vi "Thermochiller_NEWEST.vi"() -> ()   [LabVIEW 2016]
uses:
  <vilib>/Instr/_visa.llb/VISA Configure Serial Port (Instr).vi
panel:
  in  "flow control (0:none)":u16(ring) items=["None", "XON/XOFF", "RTS/CTS", "XON/XOFF & RTS/CTS", "DTR/DSR", "XON/XOFF & DTR/DSR"]
  in  "stop bits (10: 1 bit)":u16(ring)=10 items=["1.0"=10, "1.5"=15, "2.0"=20]
  in  "parity (0:none)":enum16{"None", "Odd", "Even", "Mark", "Space"}(ring)
  in  "data bits (8)":u16=8
  in  "VISA resource name":refnum<visa-resource-name>
  out "Temperature 3":cluster{"Y":dbl[], "Y":dbl[]}[](graph)
  in  "Exit":bool
  in  "Graph":bool
  out "Read Current T":string
  out "Temperature 2":dbl(knob) scale=0.0..50.0
  out "T, C":dbl
  in  "Set T Button":bool
  in  "Set T":dbl
  # "SMC THERMOCHILLER HRS -"
  # "Конфигурация оборудования"
  # "Установка температуры"
  # "Текущая температура"
  # "(c) 2021 Vladimir Z Inc.  ALL RIGHTS RESERVED."
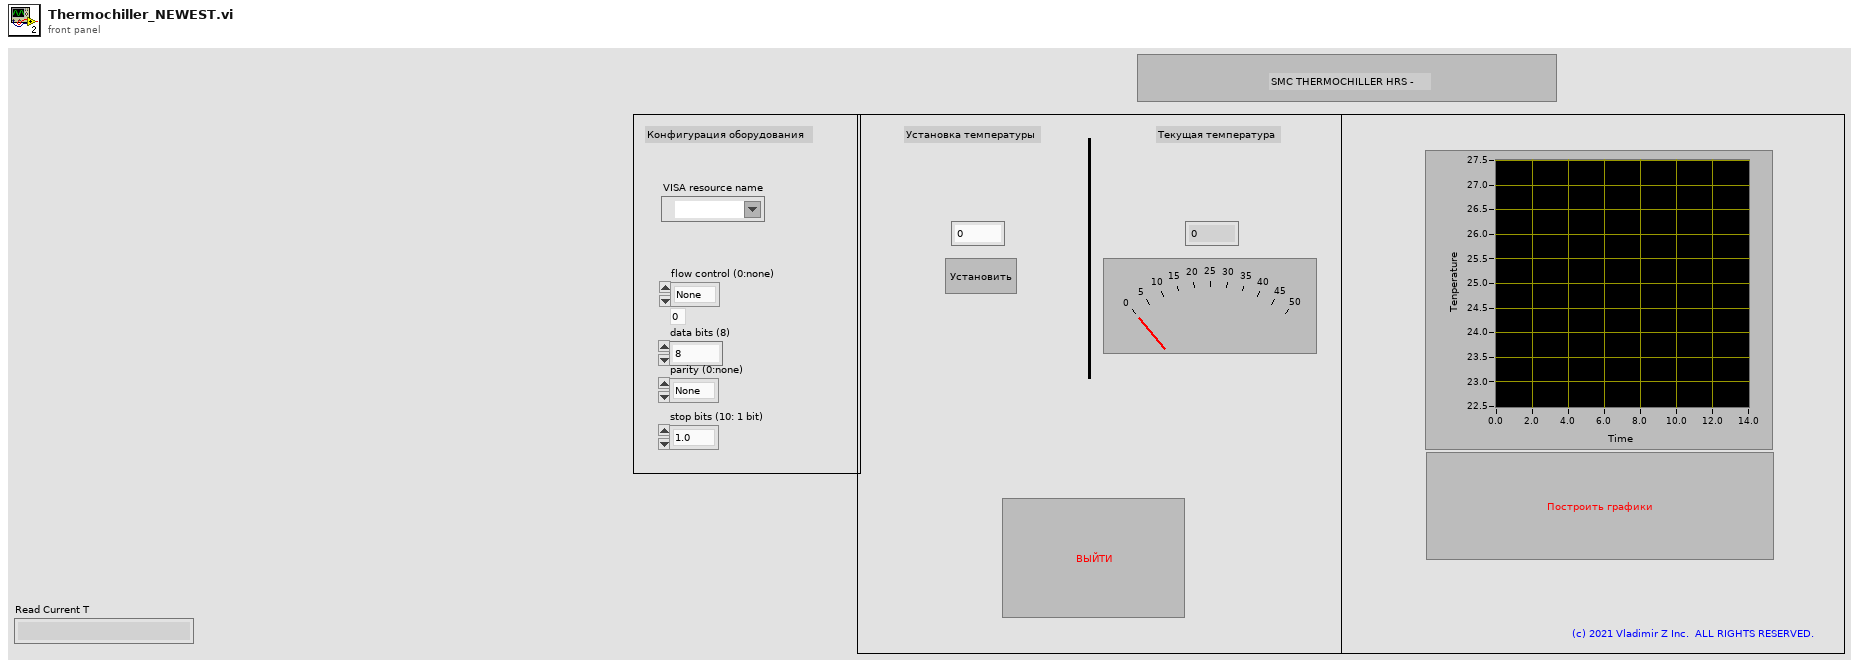
[diagram p1: front panel]
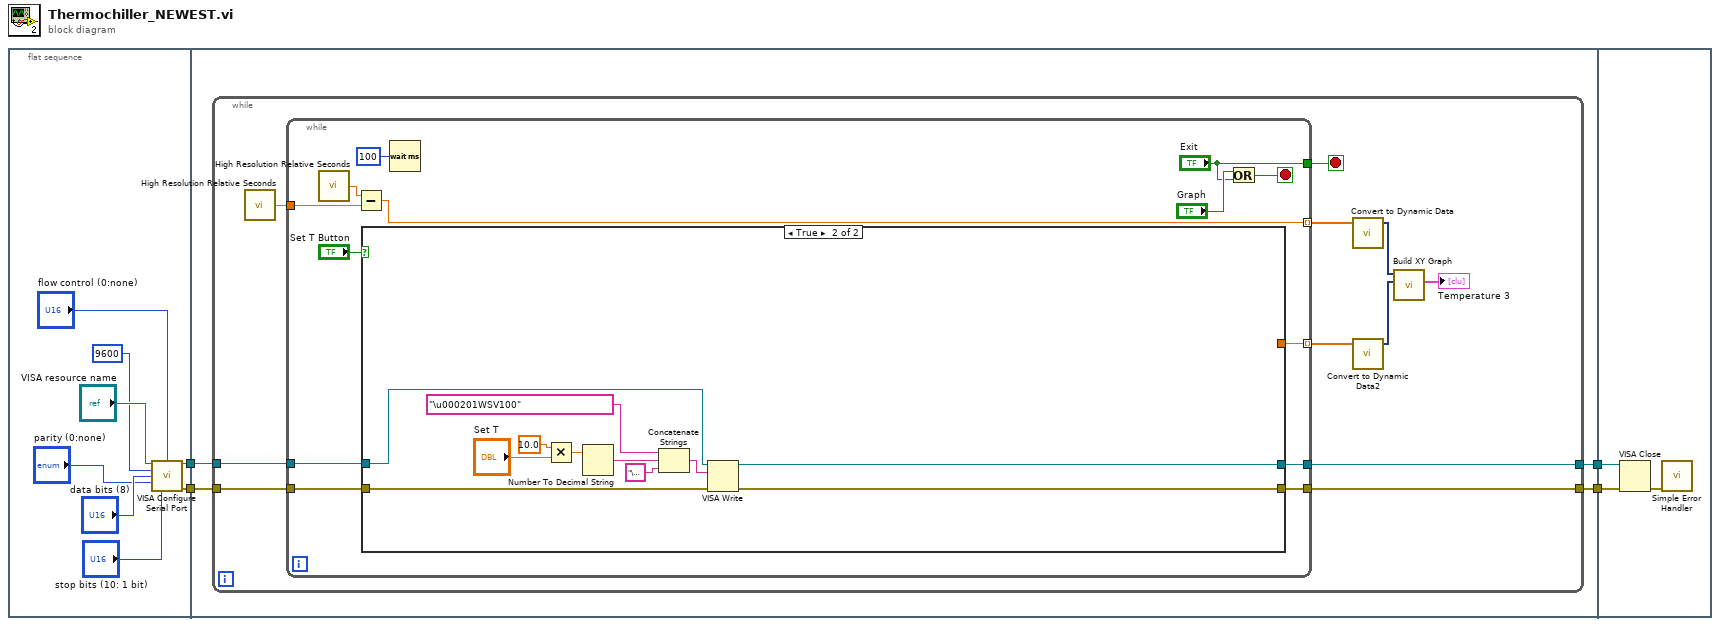
[diagram p0: block diagram]
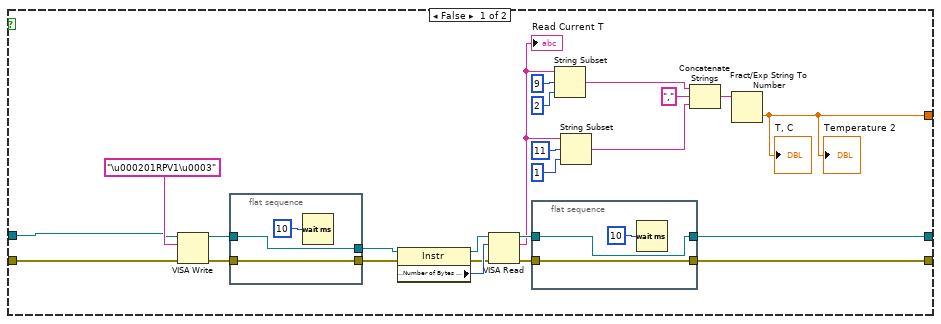
[diagram p2: hidden frame]
diagram:
  n1 = flat-sequence {
    tunnel: [w8] -> w4
    tunnel: [w7] -> w3
    tunnel: w4 -> [w16]
    tunnel: w3 -> [w15]
    tunnel: [w14] -> w2
    tunnel: [w13] -> w1
    tunnel: w2 -> [w84]
    tunnel: w1 -> [w83]
    frame #0 {
      n2 = call-poly "VISA Configure Serial Port"("VISA resource name"="VISA resource name", "baud rate (9600)"=u32 9600, "data bits (8)"="data bits (8)", "parity (0:none)"="parity (0:none)", "stop bits (10: 1 bit)"="stop bits (10: 1 bit)", "flow control (0:none)"="flow control (0:none)") -> ("VISA resource name out"=w8:refnum<visa-resource-name>, "error out"=w7:errorcluster)  [unwired: 8 in]
    }
    frame #1 {
      n3 = while {
        tunnel: w16 -> [w20]
        tunnel: w15 -> [w19]
        tunnel: [w18] -> w14
        tunnel: [w17] -> w13
        stop <- w21 stop-if-true
        n4 = call <vilib>:"High Resolution Relative Seconds.vi"() -> ("relative seconds"=w27:dbl)
        n5 = while {
          tunnel: w27 -> [w38]
          tunnel: [w36] -> w25 mode=indexing
          tunnel: [w35] -> w23 mode=indexing
          tunnel: ["Exit"] -> w21
          tunnel: w20 -> [w32]
          tunnel: w19 -> [w31]
          tunnel: [w30] -> w18
          tunnel: [w29] -> w17
          stop <- w34 stop-if-true
          n6 = call <vilib>:"High Resolution Relative Seconds.vi"() -> ("relative seconds"=w37:dbl)
          n7 = Subtract(x=w37, y=w38) -> (x-y=w36:dbl)
          n8 = case shown="True" "Set T Button" {
            tunnel: [w45 _] -> w35
            tunnel: w32 -> [w44 w74]
            tunnel: w31 -> [w43 w73]
            tunnel: [w42 w72] -> w30
            tunnel: [w41 w71] -> w29
            frame False {
              n9 = VISA Write(VISA resource name=w44, write buffer="\u000201RPV1\u0003", error in (no error)=w43) -> (VISA resource name out=w48:refnum<visa-resource-name>, error out=w49:errorcluster)  [unwired: 1 out]
              n10 = flat-sequence {
                tunnel: [w68] -> w64
                tunnel: [w69] -> w63
                tunnel: w49 -> [w69]
                tunnel: w48 -> [w68]
                frame #0 {
                  n11 = Wait (ms)(milliseconds to wait=u32 10) -> ()  [unwired: 1 out]
                }
              }
              n12 = property class="Instr"(reference=w64, error in=w63) -> (reference out=w62:refnum<visa-resource-name>, error out=w60:errorcluster, "Serial Settings:Number of Bytes at Serial Port"=w61:u32)
              n13 = VISA Read(VISA resource name=w62, byte count=w61, error in (no error)=w60) -> (VISA resource name out=w58:refnum<visa-resource-name>, read buffer=w55:string, error out=w59:errorcluster)  [unwired: 1 out]
              "Read Current T" <- w55
              n14 = flat-sequence {
                tunnel: [w65] -> w42
                tunnel: [w66] -> w41
                tunnel: w59 -> [w66]
                tunnel: w58 -> [w65]
                frame #0 {
                  n15 = Wait (ms)(milliseconds to wait=u32 10) -> ()  [unwired: 1 out]
                }
              }
              n16 = String Subset(string=w55, offset (0)=9, length (rest)=2 ("length (rest)")) -> (substring=w52:string)
              n17 = String Subset(string=w55, offset (0)=11, length (rest)=1 ("length (rest)")) -> (substring=w51:string)
              n18 = Concatenate Strings(w52, "," ("string"), w51) -> (w46:string)
              n19 = Fract/Exp String To Number(string=w46) -> (number=w45:dbl)  [unwired: 3 in, 1 out]
              "Temperature 2" <- w45
              "T, C" <- w45
            }
            frame True {
              n20 = Multiply(x=10.0, y="Set T") -> (x*y=w76:dbl)
              n21 = Number To Decimal String(number=w76) -> (decimal integer string=w78:string)  [unwired: 1 in]
              n22 = Concatenate Strings("\u000201WSV100" ("string"), w78, "\u0003" ("string")) -> (w79:string)
              n23 = VISA Write(VISA resource name=w74, write buffer=w79, error in (no error)=w73) -> (VISA resource name out=w72:refnum<visa-resource-name>, error out=w71:errorcluster)  [unwired: 1 out]
            }
          }
          n24 = Wait (ms)(milliseconds to wait=u32 100) -> ()  [unwired: 1 out]
          n25 = Or(x="Graph", y="Exit") -> (x .or. y?=w34:bool)
        }
        n26 = call "Convert to Dynamic Data"("Array"=w25) -> ("Dynamic Data Type"=w24:dynamicdata)  [unwired: 3 in]
        n27 = call "Convert to Dynamic Data2"("Array"=w23) -> ("Dynamic Data Type"=w22:dynamicdata)  [unwired: 3 in]
        n28 = call "Build XY Graph"("Y Input"=w22, "X Input"=w24) -> ("XY Graph"=→"Temperature 3":cluster{"X":dbl[], "Y":dbl[]}[])  [unwired: 8 in, 1 out]
      }
    }
    frame #2 {
      n29 = VISA Close(VISA resource name=w84, error in (no error)=w83) -> (error out=w82:errorcluster)
      n30 = call <vilib>:"Simple Error Handler.vi"("error in (no error)"=w82) -> ()  [unwired: 4 in, 5 out]
    }
  }
